vi "Motic Set RGB Gain Index.vi"(7 "b":i32, 8 "error in (no error)":errorcluster, 9 "g":i32, 10 "r":i32, 11 "camera":i32) -> (0 "error out":errorcluster, 3 "camera out":i32)   [LabVIEW 2012, in "MoticApi.lvlib"]
doc: "MOTICAPI bool Motic_SetRGBGainIndex(MUCam_Handle camera, int r, int g, int b);"
uses:
  MoticApi.lvlib
  MoticApi.dll
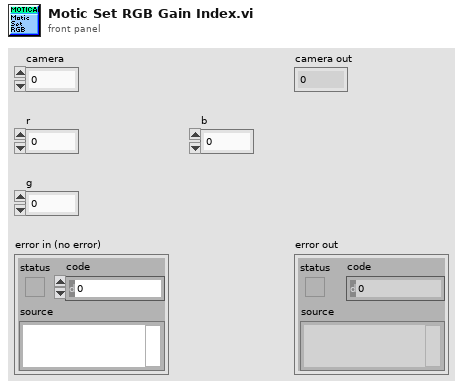
[diagram p1: front panel]
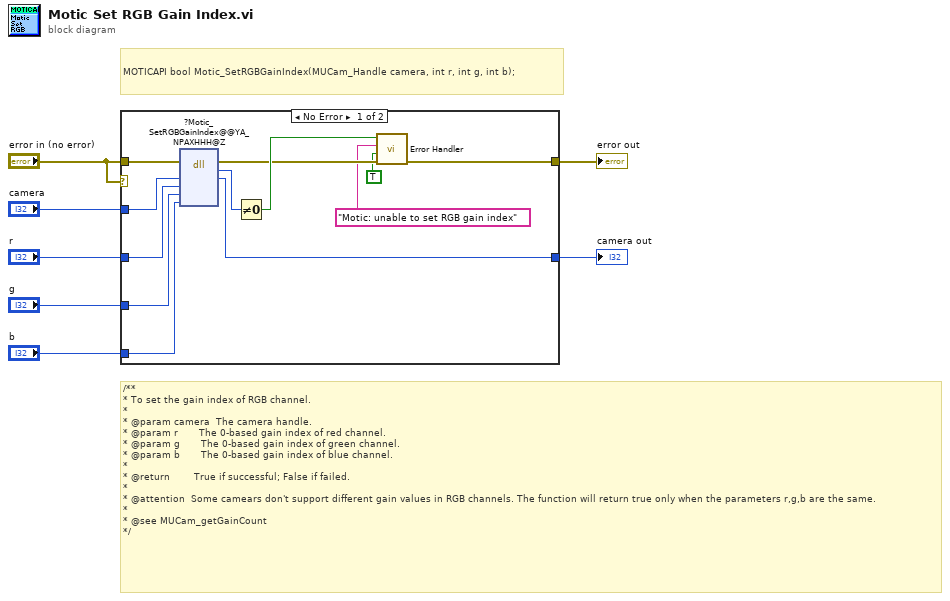
[diagram p0: block diagram]
diagram:
  # "/**\n* To set the gain index of RGB channel.\n*\n* @param camera  The camera handle.\n* @param r       The 0-based gain index of red channel.\n* @param g       The 0-based gain index of green channel.\n* @param b       The 0-based gain index of blue channel.\n*\n* @return        True if successful; False if failed.\n*\n* @attention  Some camears don't support different gain values in RGB channels. The function will return true only when the parameters r,g,b are the same.\n*\n* @see MUCam_getGainCount\n*/"
  # "MOTICAPI bool Motic_SetRGBGainIndex(MUCam_Handle camera, int r, int g, int b);"
  n1 = case shown="No Error" "error in (no error)" {
    tunnel: "camera" -> [w18 w20]
    tunnel: [w17 w20] -> w6
    tunnel: "r" -> [w16 _]
    tunnel: "g" -> [w15 _]
    tunnel: "b" -> [w14 _]
    tunnel: "error in (no error)" -> [w13 w21]
    tunnel: [w10 w21] -> w2
    frame No Error {
      n2 = dll-call lib="C:/Users/TTS-Digital/Desktop/MoticApi/MoticApi_git/MoticApi/MoticApi.*" fn="?Motic_SetRGBGainIndex@@YA_NPAXHHH@Z"(error in=w13, "camera"=w18, "r"=w16, "g"=w15, "b"=w14) -> (error out=w11:errorcluster, w19:u8, "camera"=w17:i32)  [unwired: 5 in, 1 out]
      n3 = Not Equal To 0?(x=w19) -> (x != 0?=w12:bool)
      n4 = call "Error Handler.vi"("error in (no error)"=w11, "Is warning?"=TRUE, "Error message"="Motic: unable to set RGB gain index", "Function return"=w12) -> ("error out"=w10:errorcluster)  [unwired: 7 in]
    }
    frame Error {
    }
  }
  "camera out" <- w6
  "error out" <- w2
